vi "DatatoGraphNHR.vi"(0 "NHRDC 2":refnum<vi>, 5 "t0":timestamp, 7 "Data":variant, 9 "PlotYAxis":u32[](array[numeric]), 11 "error in (no error)":errorcluster) -> (4 "WaveformArray":waveform(dbl)[](array[waveform]), 6 "Incorrect DataType?":bool, 15 "error out":errorcluster)   [LabVIEW 2018, in "AcPwrModule.lvlib"]
uses:
  AcPwrModule.lvlib
  AcPwrPlugins/AcPwrBaseClass/TypeDefs/BaseMeasurements.ctl
  AcPwrPlugins/ChromaAcLoad/TypeDefs/MeasurementType.ctl
  AcPwrPlugins/ChromaAcLoad/ChromaAcLoad.lvclass
  AcPwrPlugins/AcPwrBaseClass/AcPwrBase.lvclass
panel:
  out "Measurement":i32(ring)=1 items=["Voltage"=1, "Positive Peak Voltage"=2, "Positive Peak Voltage Last Fetch"=4, "Negative Peak Voltage"=8, "Negative Peak Voltage Last Fetch"=16, "Current"=32, "Positive Peak Current"=64, "Positive Peak Current Last Fetch"=128, "Negative Peak Current"=256, "Negative Peak Current Last Fetch"=512, "Power"=1024, "Positive Peak Power"=2048, "Positive Peak Power Last Fetch"=4096, "Negative Peak Power"=8192, "Negative Peak Power Last Fetch"=16384, "Timestamp"=32768, "Charge Time"=65536, "Discharge Time"=131072, "Amp Hour"=262144, "Amp Hour Time"=524288, "Amp Hour Charge"=1048576, "Amp Hour Discharge"=2097152, "Kilo Watt Hour"=4194304, "Kilo Watt Hour Time"=8388608, "Kilo Watt Hour Charge"=16777216, "Kilo Watt Hour Discharge"=33554432, "UUT Temperature"=67108864]
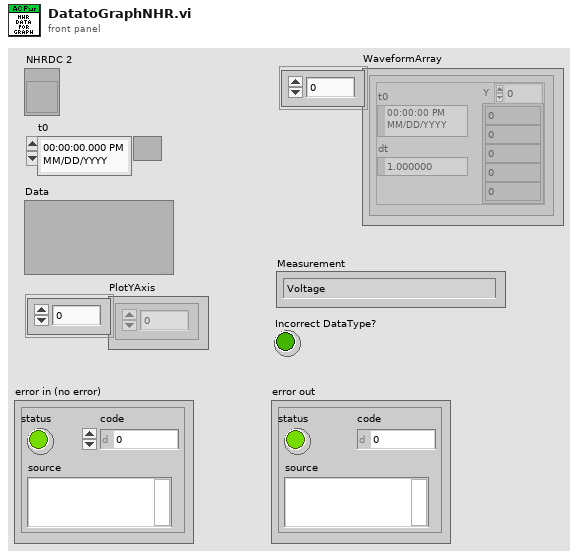
[diagram p1: front panel]
types:
  T1 = typedef "AcPwrPlugins.lvlib/AcPwrBase.lvclass/BaseMeasurements.ctl" = cluster{"Handle":string, "Name":string, "Enabled":bool, "Measurement Value":dbl, "btnMeasFetch":bool, "Chroma Hold Peak Current Measurement":bool, "Chroma Measurement Type":T2, "Chroma Protection Status String":string, "NHRDC Fetch Method":i32, "NHRDC Fetch Time (s)":sgl, "NHRDC Measurement Type":i32, "NHRGridSim Measurement Type ":enum16{"Average Current", "Max Current", "Min Current", "Average Voltage", "Max Voltage", "Min Voltage", "Average True Power", "Max True Power", "Min True Power", "Average Apparent Power", "Max Apparent Power", "Min Apparent Power", "Power Factor", "Crest Factor"}, "NHRGridSim Phase ":i32, "PPS Measurement Type ":enum16{"Voltage RMS L-N", "Voltage RMS L-L", "Frequency", "Current RMS", "Current Peak", "Crest Factor", "Power Factor", "Power VA", "Real Power"}, "PPS Channel Name":enum16{"A", "B", "C"}}[]
  T2 = typedef "AcPwrPlugins.lvlib/ChromaAcLoad.lvclass/MeasurementType.ctl" = enum16{"Voltage (Vrms or V)", "Current (Arms or A)", "Power (W)", "Peak Voltage (V)", "Peak Current (A)", "Peak Power (W)", "Frequency (Hz)", "Resistance (Ohms)", "Voltage Overshoot (V)", "Positive Peak Current (A)", "Voltage Undershoot (V)", "Negative Peak Current (A)", "Apparent Power (VA)", "Reacitive Power (VAR)", "Voltage THD", "Power Factor", "Current's Crest Factor"}
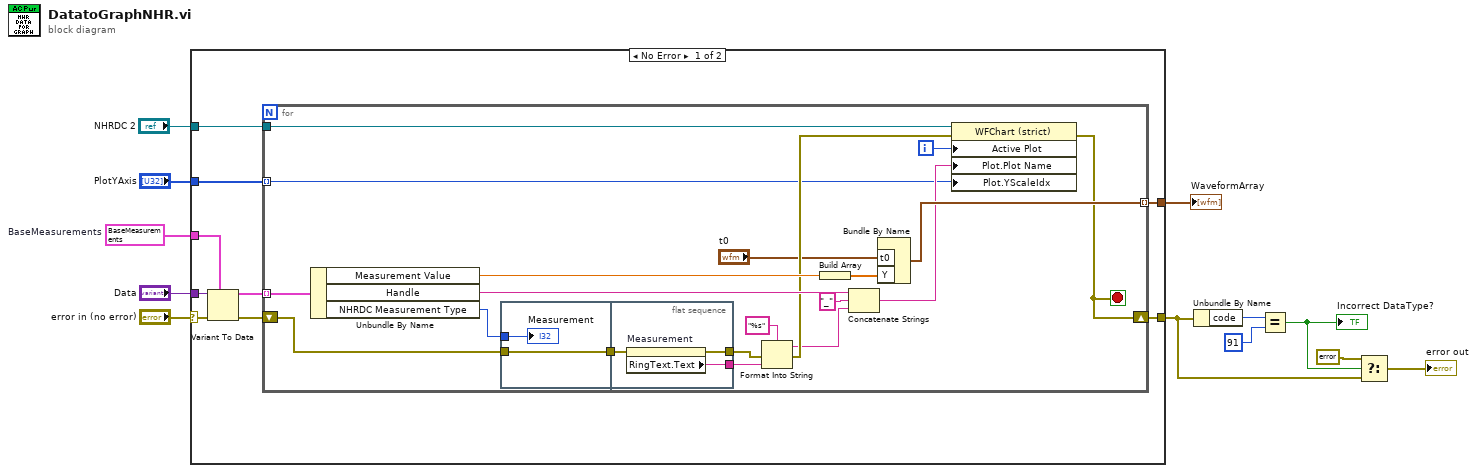
[diagram p0: block diagram]
diagram:
  w1 = T1 [{"Handle"="", "Name"="", "Enabled"=FALSE, "Measurement Value"=0.0, "btnMeasFetch"=FALSE, "Chroma Hold Peak Current Measurement"=FALSE, "Chroma Measurement Type"=enum."Voltage (Vrms or V)", "Chroma Protection Status String"="", "NHRDC Fetch Method"=0, "NHRDC Fetch Time (s)"=0.0, "NHRDC Measurement Type"=1, "NHRGridSim Measurement Type "=enum."Average Current", "NHRGridSim Phase "=0, "PPS Measurement Type "=enum."Voltage RMS L-N", "PPS Channel Name"=enum."B"}]  # BaseMeasurements
  n1 = case shown="No Error" "error in (no error)" {
    selector: "error in (no error)" -> [w15 w47]
    tunnel: [w21 _] -> w2
    tunnel: w1 -> [w20 _]
    tunnel: "Data" -> [w19 _]
    tunnel: [w18 w47] -> w4
    tunnel: "NHRDC 2" -> [w17 _]
    tunnel: "PlotYAxis" -> [w16 _]
    frame No Error {
      n2 = Variant To Data(error in=w15, type=w20, Variant=w19) -> (data=w13:T1, error out=w14:errorcluster)
      n3 = for {
        shift-right: [w24] -> w18
        shift-left: w14 -> [w29]
        tunnel: w13 -> [w41] mode=indexing
        tunnel: [w40] -> w21 mode=indexing
        tunnel: w17 -> [w26]
        tunnel: w16 -> [w25] mode=indexing
        i -> [w39]
        stop <- w24 stop-if-true
        n4 = Unbundle By Name(w41) -> ("Measurement Value"=w38:dbl, "Handle"=w36:string, "NHRDC Measurement Type"=w23:i32)
        n5 = flat-sequence {
          tunnel: w29 -> [w43]
          tunnel: [w43] -> w27
          tunnel: w23 -> [w42]
          tunnel: [w46] -> w30
          tunnel: [w44] -> w28
          tunnel: w27 -> [w45]
          frame #0 {
            "Measurement" <- w42
          }
          frame #1 {
            n6 = property on="Measurement" class="Ring (strict)"(error in=w45) -> (error out=w44:errorcluster, "RingText.Text"=w46:string)  [unwired: 1 in, 1 out]
          }
        }
        n7 = Format Into String(format string="%s", error in=w28, w30) -> (resulting string=w33:string, error out=w34:errorcluster)  [unwired: 1 in]
        n8 = Build Array(w38) -> (w37:dbl[])
        n9 = Concatenate Strings(w36, "_" ("string"), w33) -> (w32:string)
        n10 = Bundle By Name("t0"="t0", "Y"=w37) -> (w40:waveform(dbl))  [unwired: 1 in]
        n11 = property on="Property Node" class="WFChart (strict)"(reference=w26, error in=w34, "Active Plot"=w39, "Plot.Plot Name"=w32, "Plot.YScaleIdx"=w25) -> (error out=w24:errorcluster)  [unwired: 1 out]
      }
    }
    frame Error {
    }
  }
  "WaveformArray" <- w2
  n12 = Unbundle By Name(w4) -> ("code"=w9:i32)
  n13 = Equal?(x=w9, y=91) -> (x = y?=w5:bool)
  "Incorrect DataType?" <- w5
  n14 = Select(t=errorcluster {"status"=FALSE, "code"=0, "source"=""} ("error IO"), s=w5, f=w4) -> (s? t:f=→"error out":errorcluster)
